vi "Set Status Channel.vi"(7 "measure call context in":refnum<class "Measure Call Context.lvclass">, 9 "trigger":u32(ring), 10 "channels":u32(ring)) -> ()   [LabVIEW 2024, in "DSA_CFG_ACQ.lvlib"]
uses:
  DSA_CFG_ACQ.lvlib
  <vilib>/Plug-In SDKs/Measurements/Measure Call Context/Measure Call Context.lvclass
  Measurement Results.ctl
  Dynamic Signal Acquisition (Interactive).lvlib
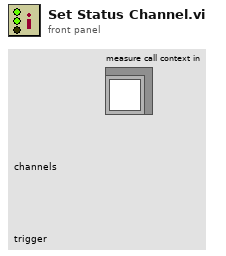
[diagram p1: front panel]
types:
  T1 = typedef "Dynamic Signal Acquisition (Interactive).lvlib/Measurement Results.ctl" = cluster{"status":bool, "DAQ channels":u32, "DAQ trigger":u32, "measurements":bool, "packed waveforms":dbl[][], "packed spectra":dbl[][], "spectra info":string[][], "averages":dbl}
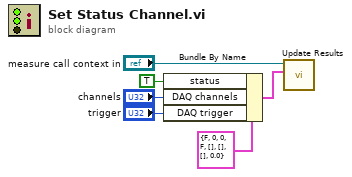
[diagram p0: block diagram]
diagram:
  n1 = Bundle By Name(cluster=T1 {"status"=FALSE, "DAQ channels"=0, "DAQ trigger"=0, "measurements"=FALSE, "packed waveforms"=[], "packed spectra"=[], "spectra info"=[], "averages"=0.0} ("Measurement Results"), "status"=TRUE, "DAQ channels"="channels", "DAQ trigger"="trigger") -> (w1:T1)
  n2 = call <vilib>:"Update Results.vi"("measurement results"=w1, "measure call context in"="measure call context in") -> ()  [unwired: 8 in, 2 out]
